vi "Periodic Tasks.vi"(8 "error in":errorcluster) -> ()   [LabVIEW 2013]
doc: "This VI runs in parallel to other tasks. It can contain as many user-defined periodic loops as you need. These can carry out PID or other sorts of timed response."
uses:
  <vilib>/Rock Robotics/SystemInterfaces/Utilities/FPGA_UtilitiesLED Source.ctl
  <vilib>/Rock Robotics/SystemInterfaces/Utilities/FPGA_UtilitiesLED State.ctl
  <vilib>/Rock Robotics/WPI/Compressor/WPI_CompressorGetSetRefNum.vi
  Robot Global Data.vi
panel:
  out "Gyro":dbl
  out "Gyro Gauge":dbl(knob) scale=0.0..10.0
  out "Encoder Alarm Statuses":string[](array[string])
  out "Directions":string[](array[string])
  out "Velocities":dbl[](array[numeric])
  out "Encoder Distances":dbl[](array[numeric])
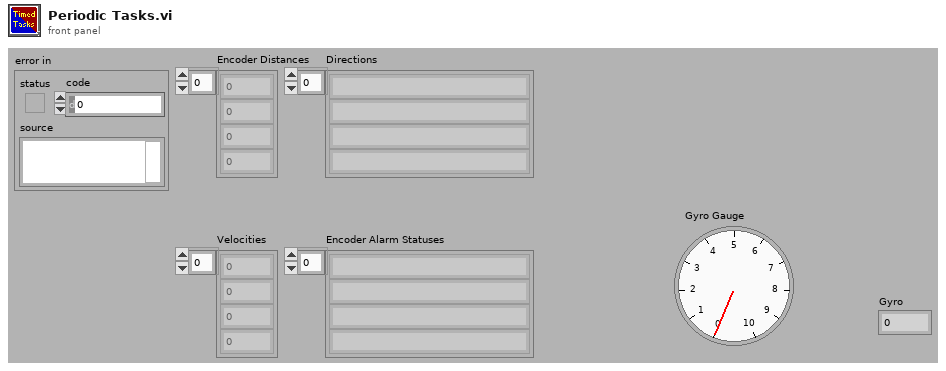
[diagram p1: front panel]
types:
  T1 = typedef "FPGA_UtilitiesLED State.ctl" = enum16{"Off", "On", "Toggle"}
  T2 = typedef "FPGA_UtilitiesLED Source.ctl" = enum16{"User LED", "FPGA LED"}
  T3 = typedef "WPI_GyroDevRef.ctl" = cluster{"DevStatus":errorcluster, "Analog Module":T4, "Analog Channel":T5, "Offset":dbl, "Gain (VoltsPerDegree/Second)":dbl}
  T4 = typedef "FPGA_TypedefAnalogModule.ctl" = enum16{"Analog Module 1", "Analog Module 2"}
  T5 = typedef "FPGA_AIChannel.ctl" = enum8{"AI 1", "AI 2", "AI 3", "AI 4", "AI 5", "AI 6", "AI 7", "AI 8", "Invalid"}
  T6 = typedef "WPI_CompressorDevRef.ctl" = cluster{"DevStatus":errorcluster, "DigitalInputDevRef":T7, "RelayDevRef":T10}
  T7 = typedef "WPI_DigitalInputDevRef.ctl" = cluster{"DevStatus":errorcluster, "DIO Channel":T8, "Digital Module":T9}
  T8 = typedef "FPGA_DIOChannel.ctl" = enum8{"DIO 1", "DIO 2", "DIO 3", "DIO 4", "DIO 5", "DIO 6", "DIO 7", "DIO 8", "DIO 9", "DIO 10", "DIO 11", "DIO 12", "DIO 13", "DIO 14", "Invalid"}
  T9 = typedef "FPGA_TypedefDigitalModule.ctl" = enum16{"Digital Module 1", "Digital Module 2"}
  T10 = typedef "WPI_RelayDevRef.ctl" = cluster{"DevStatus":errorcluster, "Relay Channel":T11, "Digital Module":T9, "Relay Direction":T12}
  T11 = typedef "FPGA_DIORelayChannel.ctl" = enum8{"Relay 1", "Relay 2", "Relay 3", "Relay 4", "Relay 5", "Relay 6", "Relay 7", "Relay 8", "Invalid"}
  T12 = typedef "WPI_RelayDirection.ctl" = enum16{"Both directions", "Forward only", "Reverse only"}
  T13 = typedef "WPI_EncoderDevRef.ctl" = cluster{"DevStatus":errorcluster, "EncoderIndex":T14, "CounterIndex":T15, "DistancePerCount":dbl, "Decoding Type":T16}
  T14 = typedef "FPGA_EncoderIdx.ctl" = enum8{"Enc 0", "Enc 1", "Enc 2", "Enc 3", "Invalid"}
  T15 = typedef "FPGA_CounterCtrSystemIndex.ctl" = enum8{"Ctr 0", "Ctr 1", "Ctr 2", "Ctr 3", "Ctr 4", "Ctr 5", "Ctr 6", "Ctr 7", "Invalid"}
  T16 = typedef "WPI_EncoderType.ctl" = enum16{"1x", "2x", "4x"}
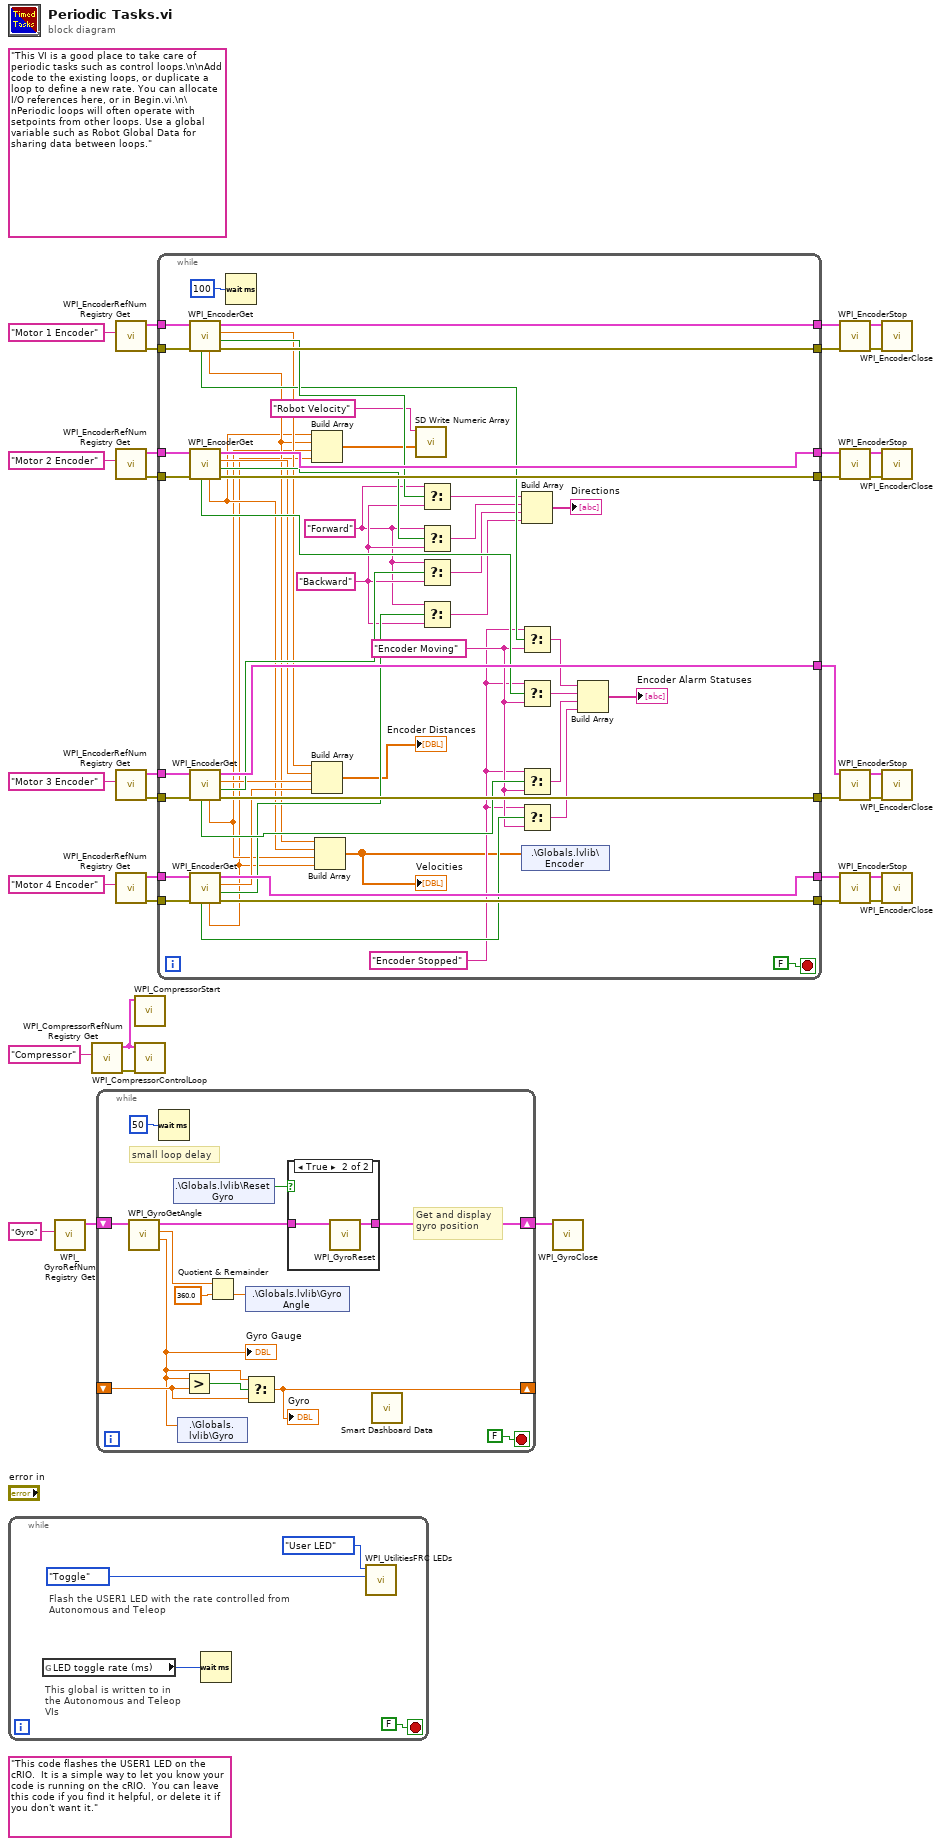
[diagram p0: block diagram]
diagram:
  (unwired) "This code flashes the USER1 LED on the cRIO.  It is a simple way to let you know your code is running on the cRIO.  You can leave this code if you find it helpful, or delete it if you don't want it."
  (unwired) "This VI is a good place to take care of periodic tasks such as control loops.\n\nAdd code to the existing loops, or duplicate a loop to define a new rate. You can allocate I/O references here, or in Begin.vi.\n\nPeriodic loops will often operate with setpoints from other loops. Use a global variable such as Robot Global Data for sharing data between loops."
  n1 = while {
    stop <- FALSE stop-if-true
    # "This global is written to in the Autonomous and Teleop VIs"
    # "Flash the USER1 LED with the rate controlled from Autonomous and Teleop"
    n2 = global read "Robot Global Data.vi" "LED toggle rate (ms)"() -> (w35:u32)
    n3 = Wait (ms)(milliseconds to wait=w35) -> ()  [unwired: 1 out]
    n4 = call <vilib>:"WPI_UtilitiesFRC LEDs.vi"("State"=FPGA_UtilitiesLED_State."Toggle", "LED Type"=FPGA_UtilitiesLED_Source."User LED") -> ()  [unwired: 1 in, 9 out]
  }
  n5 = call <vilib>:"WPI_GyroRefNum Registry Get.vi"("refnum name"="Gyro") -> ("GyroDevRef"=w34:T3)  [unwired: 9 in, 1 out]
  n6 = call <vilib>:"WPI_CompressorRefNum Registry Get.vi"("refnum name"="Compressor") -> ("error out"=w2:errorcluster, "CompressorDevRef"=w3:T6)  [unwired: 9 in]
  n7 = while {
    shift-right: [w46] -> w32
    shift-left: w34 -> [w48]
    shift-right: [w40] -> _
    shift-left: _ -> [w41]
    stop <- FALSE stop-if-true
    # "small loop delay"
    # "Get and display\ngyro position"
    n8 = call <vilib>:"WPI_GyroGetAngle.vi"("GyroDevRef"=w48) -> ("Angular Rate"=w39:dbl, "Angle"=w44:dbl, "GyroDevRef"=w47:T3)  [unwired: 1 in, 7 out]
    "Gyro Gauge" <- w39
    n9 = Wait (ms)(milliseconds to wait=u32 50) -> ()  [unwired: 1 out]
    n10 = shared-variable ".\\Globals.lvlib\\Reset Gyro"() -> (w45:bool)  [unwired: 1 in, 1 out]
    n11 = shared-variable ".\\Globals.lvlib\\Gyro"(w39) -> ()  [unwired: 1 in, 1 out]
    n12 = Greater?(x=w39, y=w41) -> (0:w42:bool)
    n13 = Quotient & Remainder(x=w44, y=360.0) -> (floor(x/y)=w43:dbl)  [unwired: 1 out]
    n14 = shared-variable ".\\Globals.lvlib\\Gyro Angle"(w43) -> ()  [unwired: 1 in, 1 out]
    n15 = Select(t=w39, s=w42, f=w41) -> (s? t:f=w40:dbl)
    "Gyro" <- w40
    n16 = case shown="True" w45 {
      tunnel: w47 -> [w52 w54]
      tunnel: [w52 w53] -> w46
      frame False {
      }
      frame True {
        n17 = call <vilib>:"WPI_GyroReset.vi"("GyroDevRef"=w54) -> ("GyroDevRef"=w53:T3)  [unwired: 9 in, 1 out]
      }
    }
    n18 = call "Smart Dashboard Data.vi"() -> ()  [unwired: 12 in]
  }
  n19 = call <vilib>:"WPI_EncoderRefNum Registry Get.vi"("refnum name"="Motor 1 Encoder") -> ("error out"=w30:errorcluster, "EncoderDevRef"=w31:T13)  [unwired: 9 in]
  n20 = call <vilib>:"WPI_EncoderRefNum Registry Get.vi"("refnum name"="Motor 2 Encoder") -> ("error out"=w27:errorcluster, "EncoderDevRef"=w26:T13)  [unwired: 9 in]
  n21 = call <vilib>:"WPI_EncoderRefNum Registry Get.vi"("refnum name"="Motor 3 Encoder") -> ("error out"=w24:errorcluster, "EncoderDevRef"=w25:T13)  [unwired: 9 in]
  n22 = call <vilib>:"WPI_EncoderRefNum Registry Get.vi"("refnum name"="Motor 4 Encoder") -> ("error out"=w5:errorcluster, "EncoderDevRef"=w4:T13)  [unwired: 9 in]
  n23 = call <vilib>:"WPI_CompressorStart.vi"("CompressorDevRef"=w3) -> ()  [unwired: 9 in, 2 out]
  n24 = call <vilib>:"WPI_CompressorControlLoop.vi"("error in (no error)"=w2, "CompressorDevRef"=w3) -> ()  [unwired: 10 in]
  n25 = while {
    tunnel: w31 -> [w106]
    tunnel: w30 -> [w105]
    tunnel: w27 -> [w104]
    tunnel: w26 -> [w103]
    tunnel: w25 -> [w102]
    tunnel: w24 -> [w101]
    tunnel: [w100] -> w22
    tunnel: [w99] -> w19
    tunnel: [w98] -> w15
    tunnel: [w97] -> w14
    tunnel: [w96] -> w13
    tunnel: [w95] -> w11
    tunnel: [w94] -> w10
    tunnel: [w93] -> w7
    tunnel: w5 -> [w92]
    tunnel: w4 -> [w91]
    stop <- FALSE stop-if-true
    w79 = "Backward" ("f")
    w80 = "Encoder Moving" ("f")
    w77 = "Encoder Stopped"
    w78 = "Forward"
    n26 = call <vilib>:"WPI_EncoderGet.vi"("error in (no error)"=w105, "EncoderDevRef"=w106) -> ("error out"=w98:errorcluster, "Direction"=w85:bool, "Distance"=w76:dbl, "EncoderDevRef"=w100:T13, "Rate"=w71:dbl, "Stopped"=w84:bool)  [unwired: 4 out]
    n27 = call <vilib>:"WPI_EncoderGet.vi"("error in (no error)"=w104, "EncoderDevRef"=w103) -> ("error out"=w96:errorcluster, "Direction"=w83:bool, "Distance"=w75:dbl, "EncoderDevRef"=w97:T13, "Rate"=w70:dbl, "Stopped"=w82:bool)  [unwired: 4 out]
    n28 = call <vilib>:"WPI_EncoderGet.vi"("error in (no error)"=w101, "EncoderDevRef"=w102) -> ("error out"=w95:errorcluster, "Direction"=w89:bool, "Distance"=w74:dbl, "EncoderDevRef"=w99:T13, "Rate"=w69:dbl, "Stopped"=w88:bool)  [unwired: 4 out]
    n29 = call <vilib>:"WPI_EncoderGet.vi"("error in (no error)"=w92, "EncoderDevRef"=w91) -> ("error out"=w94:errorcluster, "Direction"=w87:bool, "Distance"=w73:dbl, "EncoderDevRef"=w93:T13, "Rate"=w55:dbl, "Stopped"=w86:bool)  [unwired: 4 out]
    n30 = Wait (ms)(milliseconds to wait=u32 100) -> ()  [unwired: 1 out]
    n31 = Build Array(w70, w71, w69, w55) -> (w58:dbl[])
    n32 = Build Array(w76, w75, w74, w73) -> (→"Encoder Distances":dbl[])
    n33 = Build Array(w71, w70, w69, w55) -> (w56:dbl[])
    "Velocities" <- w56
    n34 = call <vilib>:"SD Write Numeric Array.vi"("Numeric Array"=w58, "Name"="Robot Velocity") -> ()  [unwired: 8 in, 2 out]
    n35 = Select(t=w78, s=w85, f=w79) -> (s? t:f=w68:string)
    n36 = Select(t=w78, s=w83, f=w79) -> (s? t:f=w67:string)
    n37 = Select(t=w78, s=w89, f=w79) -> (s? t:f=w66:string)
    n38 = Select(t=w78, s=w87, f=w79) -> (s? t:f=w65:string)
    n39 = Build Array(w68, w67, w66, w65) -> (→"Directions":string[])
    n40 = Select(t=w77, s=w84, f=w80) -> (s? t:f=w62:string)
    n41 = Select(t=w77, s=w82, f=w80) -> (s? t:f=w61:string)
    n42 = Select(t=w77, s=w88, f=w80) -> (s? t:f=w60:string)
    n43 = Select(t=w77, s=w86, f=w80) -> (s? t:f=w59:string)
    n44 = shared-variable ".\\Globals.lvlib\\Encoder"(w56) -> ()  [unwired: 1 in, 1 out]
    n45 = Build Array(w62, w61, w60, w59) -> (→"Encoder Alarm Statuses":string[])
  }
  n46 = call <vilib>:"WPI_GyroClose.vi"("GyroDevRef"=w32) -> ()  [unwired: 1 in, 10 out]
  n47 = call <vilib>:"WPI_EncoderStop.vi"("error in (no error)"=w15, "EncoderDevRef"=w22) -> ("error out"=w16:errorcluster, "EncoderDevRef"=w21:T13)  [unwired: 8 in]
  n48 = call <vilib>:"WPI_EncoderStop.vi"("error in (no error)"=w13, "EncoderDevRef"=w14) -> ("error out"=w12:errorcluster, "EncoderDevRef"=w20:T13)  [unwired: 8 in]
  n49 = call <vilib>:"WPI_EncoderStop.vi"("error in (no error)"=w11, "EncoderDevRef"=w19) -> ("error out"=w18:errorcluster, "EncoderDevRef"=w17:T13)  [unwired: 8 in]
  n50 = call <vilib>:"WPI_EncoderStop.vi"("error in (no error)"=w10, "EncoderDevRef"=w7) -> ("error out"=w8:errorcluster, "EncoderDevRef"=w9:T13)  [unwired: 8 in]
  n51 = call <vilib>:"WPI_EncoderClose.vi"("error in (no error)"=w16, "EncoderDevRef"=w21) -> ()  [unwired: 9 in, 1 out]
  n52 = call <vilib>:"WPI_EncoderClose.vi"("error in (no error)"=w12, "EncoderDevRef"=w20) -> ()  [unwired: 9 in, 1 out]
  n53 = call <vilib>:"WPI_EncoderClose.vi"("error in (no error)"=w18, "EncoderDevRef"=w17) -> ()  [unwired: 9 in, 1 out]
  n54 = call <vilib>:"WPI_EncoderClose.vi"("error in (no error)"=w8, "EncoderDevRef"=w9) -> ()  [unwired: 9 in, 1 out]
